vi "Find FFT Size Limit.vi"(8 "error in":errorcluster, 9 "Total Global Memory (Bytes)":i64, 10 "Reset Device?":bool, 11 "Device ID":T1) -> (0 "error out":errorcluster, 2 "FFT Execution Times (s)":dbl[](array[numeric]), 3 "N":i32)   [LabVIEW 2020, in "Get GPU Device Information.lvlib"]
uses:
  Get GPU Device Information.lvlib
  <vilib>/addons/lvgpu/lvcuda/CUDA Device (CUdevice).ctl
  <vilib>/addons/lvgpu/lvcufft/Create 1D FFT Plan.vi
  <vilib>/addons/lvgpu/lvcufft/Complex FFT (CSG).vi
  <vilib>/addons/lvgpu/lvcuda/CUDA CSG Device Ptr/Synchronize Context.vi
  <vilib>/addons/lvgpu/lvcuda.lvlib
  <vilib>/addons/lvgpu/lvcufft.lvlib
  <vilib>/addons/lvgpu/lvcuda/CUDA CSG Device Ptr/CUDA CSG Device Ptr.lvclass
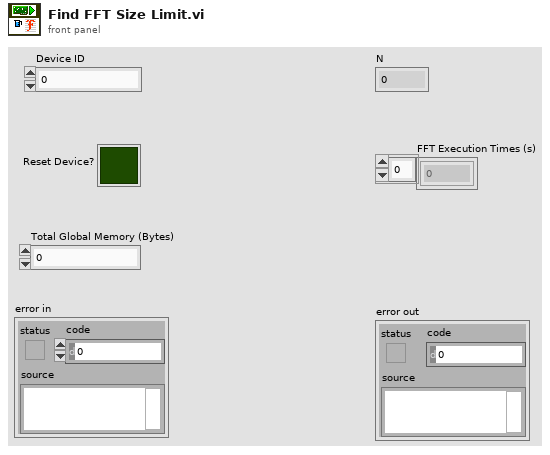
[diagram p1: front panel]
types:
  T1 = typedef "lvcuda.lvlib/CUDA Device (CUdevice).ctl" = i32
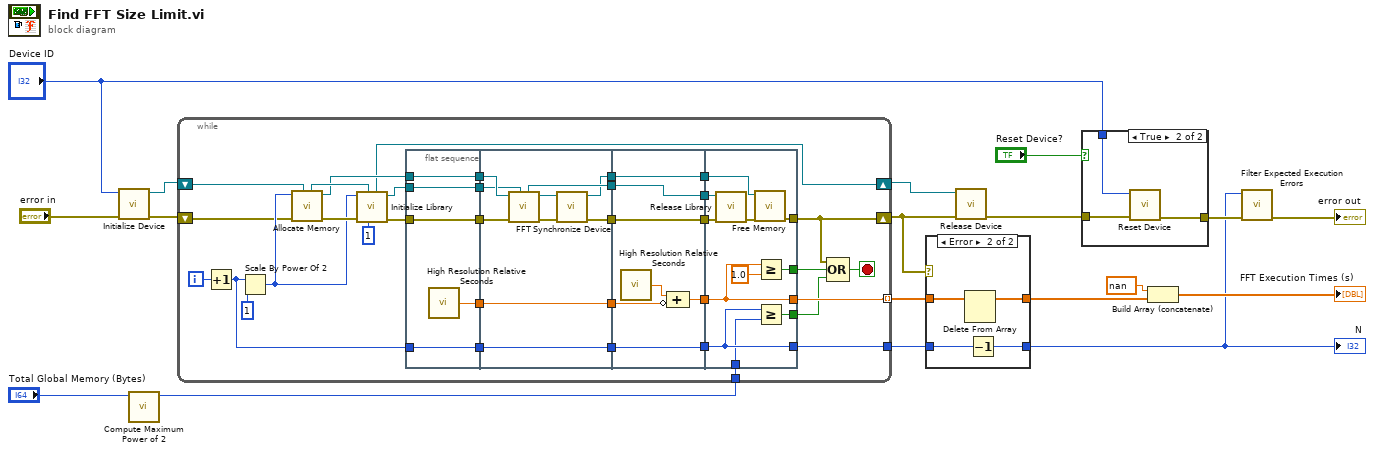
[diagram p0: block diagram]
diagram:
  n1 = call <vilib>:"Initialize Device.vi"("error in"="error in", "CUDA Device ID"="Device ID") -> ("error out"=w14:errorcluster, "CUDA Context"=w15:refnum<class "CUDA Context.lvclass">)  [unwired: 7 in, 1 out]
  n2 = call "Compute Maximum Power of 2.vi"("Total Global Memory (Bytes)"="Total Global Memory (Bytes)") -> ("Max N"=w4:i32)  [unwired: 10 in]
  n3 = while {
    shift-right: [w34] -> w16
    shift-left: w15 -> [w53]
    shift-right: [w29] -> w3
    shift-left: w14 -> [w33]
    tunnel: [w23] -> w2
    tunnel: [w31] -> w6 mode=indexing
    tunnel: w4 -> [w19]
    i -> [w21]
    stop <- w27 stop-if-true
    n4 = Increment(x=w21) -> (x+1=w20:i32)
    n5 = Scale By Power Of 2(n=w20, x=1) -> (x*2^n=w49:i32)
    n6 = call-poly <vilib>:"Allocate Memory.vi"("CUDA Context in"=w53, "error in"=w33, "size in elements"=w49) -> ("error out"=w51:errorcluster, "CUDA CSG Device Ptr out"=w44:refnum<class "CUDA CSG Device Ptr.lvclass">, "CUDA Context out"=w50:refnum<class "CUDA Context.lvclass">)  [unwired: 6 in]
    n7 = call-poly <vilib>:"Initialize Library.vi"("batch"=1, "CUDA Context in"=w50, "error in"=w51, "size"=w49) -> ("error out"=w32:errorcluster, "CUFFT Handle"=w39:refnum<class "CUFFT Handle.lvclass">, "CUDA Context out"=w34:refnum<class "CUDA Context.lvclass">)  [unwired: 4 in, 1 out]
    n8 = flat-sequence {
      tunnel: w32 -> [w56]
      tunnel: [w58] -> w47
      tunnel: [w57] -> w45
      tunnel: w44 -> [w57]
      tunnel: [w56] -> w43
      tunnel: [w55] -> w40
      tunnel: w39 -> [w55]
      tunnel: w20 -> [w54]
      tunnel: [w54] -> w24
      tunnel: w47 -> [w68]
      tunnel: [w68] -> w46
      tunnel: w45 -> [w67]
      tunnel: w43 -> [w66]
      tunnel: [w63] -> w41
      tunnel: w40 -> [w65]
      tunnel: [w61] -> w37
      tunnel: [w60] -> w35
      tunnel: [w59] -> w25
      tunnel: w24 -> [w59]
      tunnel: w46 -> [w75]
      tunnel: [w73] -> w42
      tunnel: w41 -> [w73]
      tunnel: [w72] -> w38
      tunnel: w37 -> [w72]
      tunnel: [w71] -> w36
      tunnel: w35 -> [w71]
      tunnel: [w70] -> w30
      tunnel: [w69] -> w26
      tunnel: w25 -> [w69]
      tunnel: w42 -> [w86]
      tunnel: w38 -> [w85]
      tunnel: w36 -> [w83]
      tunnel: [w82] -> w29
      tunnel: [w81] -> w31
      tunnel: w30 -> [w81]
      tunnel: [w79] -> w28
      tunnel: w26 -> [w78]
      tunnel: [w78] -> w23
      tunnel: [w77] -> w22
      tunnel: w19 -> [w76]
      frame #0 {
        n9 = call <vilib>:"High Resolution Relative Seconds.vi"() -> ("relative seconds"=w58:dbl)
      }
      frame #1 {
        n10 = call-poly <vilib>:"FFT.vi"("CUFFT Handle in"=w65, "error in"=w66, "signals in"=w67) -> ("error out"=w64:errorcluster, "spectrums out"=w62:refnum<class "CUDA CSG Device Ptr.lvclass">, "CUFFT Handle out"=w61:refnum<class "CUFFT Handle.lvclass">)  [unwired: 6 in]
        n11 = call-poly <vilib>:"Synchronize Device.vi"("error in"=w64, "CUDA CSG Device Ptr in"=w62) -> ("error out"=w63:errorcluster, "CUDA CSG Device Ptr out"=w60:refnum<class "CUDA CSG Device Ptr.lvclass">)  [unwired: 8 in]
      }
      frame #2 {
        n12 = call <vilib>:"High Resolution Relative Seconds.vi"() -> ("relative seconds"=w74:dbl)
        n13 = Compound Arithmetic op=ADD(w74, invert w75) -> (w70:dbl)
      }
      frame #3 {
        n14 = call <vilib>:"Release Library.vi"("error in"=w86, "CUFFT Handle in"=w85) -> ("error out"=w84:errorcluster)  [unwired: 9 in]
        n15 = call-poly <vilib>:"Free Memory.vi"("error in"=w84, "CUDA CSG Device Ptr in"=w83) -> ("error out"=w82:errorcluster)  [unwired: 9 in]
        n16 = Greater Or Equal?(x=w81, y=1.0) -> (x >= y?=w79:bool)
        n17 = Greater Or Equal?(x=w78, y=w76) -> (x >= y?=w77:bool)
      }
    }
    n18 = Compound Arithmetic op=OR(w29, w28, w22) -> (w27:bool)
  }
  n19 = case shown="Error" w3 {
    tunnel: [w88 w92] -> w9
    tunnel: w6 -> [w88 w91]
    tunnel: w2 -> [w87 w90]
    tunnel: [w87 w89] -> w1
    frame No Error {
    }
    frame Error {
      n20 = Delete From Array(array=w91) -> (array with subset deleted=w92:dbl[])  [unwired: 2 in, 1 out]
      n21 = Decrement(x=w90) -> (x-1=w89:i32)
    }
  }
  "N" <- w1
  n22 = call <vilib>:"Release Device.vi"("error in"=w3, "CUDA Context in"=w16) -> ("error out"=w17:errorcluster)  [unwired: 9 in]
  n23 = case shown="True" "Reset Device?" {
    tunnel: w17 -> [w93 w96]
    tunnel: "Device ID" -> [_ w95]
    tunnel: [w93 w94] -> w11
    frame False {
    }
    frame True {
      n24 = call <vilib>:"Reset Device.vi"("error in"=w96, "CUDA Device"=w95) -> ("error out"=w94:errorcluster)  [unwired: 9 in]
    }
  }
  n25 = Build Array (concatenate)(nan, w9) -> (→"FFT Execution Times (s)":dbl[])
  n26 = call "Filter Expected Execution Errors.vi"("error in"=w11, "N"=w1) -> ("error out"=→"error out":errorcluster)  [unwired: 9 in]
